vi "Initialize.vi"(8 "error in (no error)":errorcluster, 10 "Bus Monitor Configuration":T1) -> (0 "error out":errorcluster, 3 "Bus Monitor out":refnum<class "Bus Monitor.lvclass">)   [LabVIEW 2020, in "BCI-1553 API.lvlib" / "Bus Monitor.lvclass"]
doc: "Generates a Bus Monitor object that can be added to a Component. There may be a single Bus Monitor on a Component and nothing else. A Bus Monitor requires Filters added to it to capture any bus traffic."
uses:
  Bus Monitor.lvclass
  TypeDefs/Bus Monitor Configuration.ctl
  TypeDefs/Bus Monitor Timeout.ctl
  TypeDefs/Bus Monitor Timetag Behavior.ctl
  TypeDefs/Bus Monitor Record Requirement.ctl
  TypeDefs/Bus Monitor Timetag Configuration.ctl
  Bus Monitor.lvclass/Bus Monitor.ctl
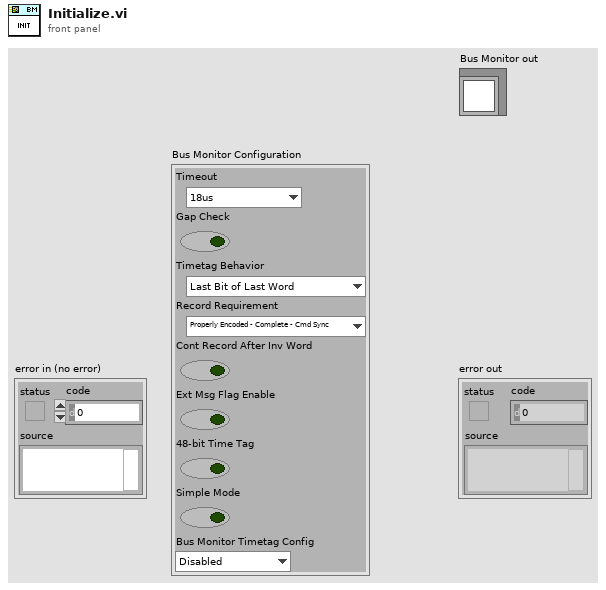
[diagram p1: front panel]
types:
  T1 = typedef "BCI-1553 API.lvlib/Bus Monitor.lvclass/Bus Monitor Configuration.ctl" = cluster{"Timeout":T2, "Gap Check":bool, "Timetag Behavior":T3, "Record Requirement":T4, "Cont Record After Inv Word":bool, "Ext Msg Flag Enable":bool, "48-bit Time Tag":bool, "Simple Mode":bool, "Bus Monitor Timetag Config":T5}
  T2 = typedef "BCI-1553 API.lvlib/Bus Monitor.lvclass/Bus Monitor Timeout.ctl" = enum16{"18us", "23us", "82us", "140us"}
  T3 = typedef "BCI-1553 API.lvlib/Bus Monitor.lvclass/Bus Monitor Timetag Behavior.ctl" = enum16{"Last Bit of Last Word", "First Bit of Command Word", "Last Bit of Command Word", "Timetag Disabled"}
  T4 = typedef "BCI-1553 API.lvlib/Bus Monitor.lvclass/Bus Monitor Record Requirement.ctl" = enum16{"Properly Encoded - Complete - Cmd Sync", "Properly Encoded - Complete - Cmd or Data Sync", "Properly Encoded Cmd Sync - At Least 2 Data Bits ", "Any Properly Encoded Sync - At Least 2 Data Bits"}
  T5 = typedef "BCI-1553 API.lvlib/Bus Monitor.lvclass/Bus Monitor Timetag Configuration.ctl" = enum16{"Disabled", "2us", "4us", "8us", "16us", "32us", "64us", "100ns"}
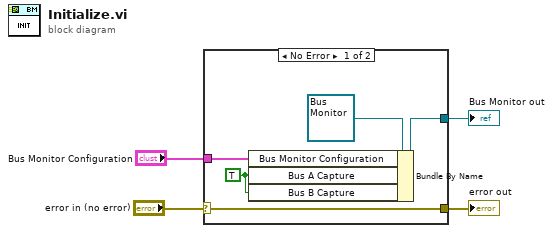
[diagram p0: block diagram]
diagram:
  n1 = case shown="No Error" "error in (no error)" {
    selector: "error in (no error)" -> [w9 w10]
    tunnel: [w9 w10] -> w3
    tunnel: "Bus Monitor Configuration" -> [w7 _]
    tunnel: [w6 _] -> w1
    frame No Error {
      w5 = TRUE ("Bus A Capture")
      n2 = Bundle By Name(cluster=refnum<class "Bus Monitor.lvclass"> refnum ("SLSC 1553 API.lvlib:Bus Monitor.lvclass"), "Bus Monitor Configuration"=w7, "Bus A Capture"=w5, "Bus B Capture"=w5) -> (w6:refnum<class "Bus Monitor.lvclass">)
    }
    frame Error {
    }
  }
  "error out" <- w3
  "Bus Monitor out" <- w1
